vi "菜单-保存.vi"(8 "error in (no error)":errorcluster caption="错误输入（无错误）", 11 "程序响应 输入":refnum<class "程序响应.lvclass">) -> (0 "error out":errorcluster caption="错误输出", 3 "程序响应 输出":refnum<class "程序响应.lvclass">)   [LabVIEW 2018, in "程序响应.lvlib" / "程序响应.lvclass"]
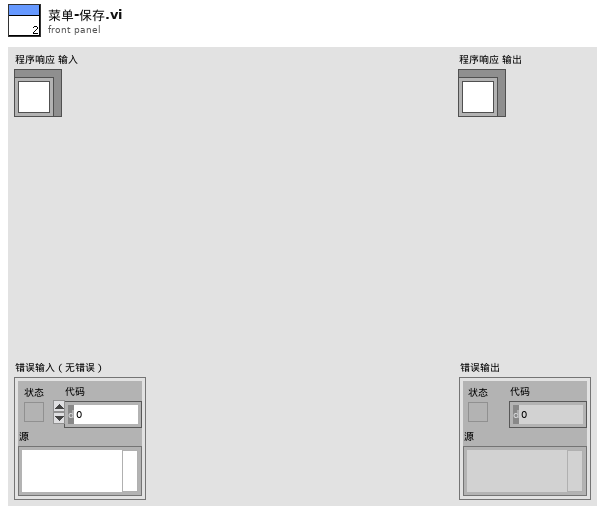
[diagram p1: front panel]
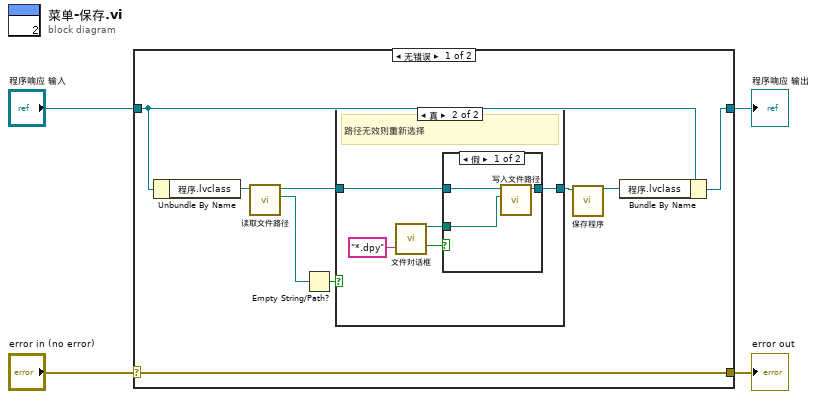
[diagram p0: block diagram]
diagram:
  n1 = case shown="无错误" "error in (no error)" {
    selector: "error in (no error)" -> [w13 w25]
    tunnel: [w13 w25] -> w3
    tunnel: [w8 w24] -> w1
    tunnel: "程序响应 输入" -> [w9 w24]
    frame No Error {
      n2 = Unbundle By Name(w9) -> ("程序.lvclass"=w12:refnum<class "程序.lvclass">)
      n3 = call-dynamic "读取文件路径.vi"("程序输入"=w12) -> ("文件路径"=w7:path, "程序输出"=w6:refnum<class "程序.lvclass">)  [unwired: 8 in, 1 out]
      n4 = Empty String/Path?(string/path=w7) -> (empty?=w11:bool)
      n5 = case shown="真" w11 {
        tunnel: w6 -> [w14 w19]
        tunnel: [w14 w18] -> w5
        frame False {
          # "路径有效则直接保存"
        }
        frame True {
          # "路径无效则重新选择"
          n6 = call "文件对话框"("pattern (all files)"="*.dpy" ("pattern label")) -> ("selected path"=w17:path, "cancelled"=w15:bool)  [unwired: 11 in, 2 out]
          n7 = case shown="假" w15 {
            tunnel: w19 -> [w22 w23]
            tunnel: [w21 w23] -> w18
            tunnel: w17 -> [w20 _]
            frame False {
              n8 = call-dynamic "写入文件路径.vi"("文件路径"=w20, "程序输入"=w22) -> ("程序输出"=w21:refnum<class "程序.lvclass">)  [unwired: 8 in, 1 out]
            }
            frame True {
            }
          }
        }
      }
      n9 = call-dynamic "保存程序.vi"("程序 输入"=w5) -> ("程序 输出"=w10:refnum<class "程序.lvclass">)  [unwired: 9 in, 1 out]
      n10 = Bundle By Name(cluster=w9, "程序.lvclass"=w10) -> (w8:refnum<class "程序响应.lvclass">)
    }
    frame Error {
    }
  }
  "error out" <- w3
  "程序响应 输出" <- w1
